vi "SwapAndFormat.vi"(4 "Mode Index":i32=2, 6 "Undo pointer":i32, 7 "Layout Ref":refnum<vi>, 8 "error in (no error)":errorcluster, 9 "Table CtlRef In":refnum<vi>, 10 "Col Array in":refnum<class "Column.lvclass">[](array[class]), 11 "OldTable Array in":T1) -> (0 "error out":errorcluster, 3 "OldTable Array out":T1)   [LabVIEW 2013]
doc: "Original use was in Un(Re)doTblChng.vi. It can also be used to apply (block-wise) changes to the table (as with PasteSafe.vi) with best choices for formatting. Input new table as 1st element in an array of cluster of table and set undo pointer to zero."
uses:
  TypeDefs/TableArray.ctl
  ColumnVIs/Column/Column.lvclass
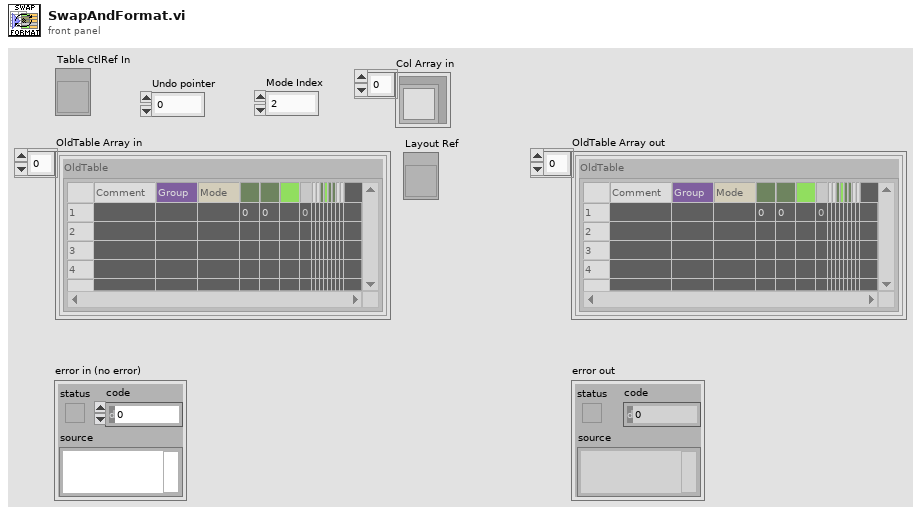
[diagram p1: front panel]
types:
  T1 = typedef "TableArray.ctl" = cluster{"OldTable":string[][]}[]
  T2 = typedef "LVRowAndColumnTypeDef.ctl" = cluster{"Row":i32, "Column":i32}
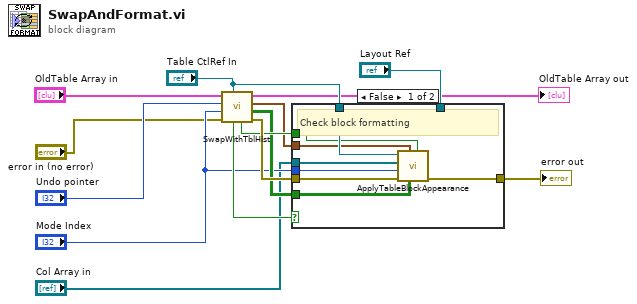
[diagram p0: block diagram]
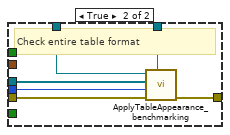
[diagram p2: hidden frame]
diagram:
  n1 = call "SwapWithTblHist.vi"("Table CtlRef In"="Table CtlRef In", "error in (no error)"="error in (no error)", "Mode Index"="Mode Index", "Undo pointer"="Undo pointer", "OldTable Array in"="OldTable Array in") -> ("error out"=w14:errorcluster, "changed? subarray"=w11:bool[][], "Change start"=w10:T2, "OldTable Array out"=→"OldTable Array out":T1, "Mode change?"=w12:bool, "Size mismatch?"=w13:bool)  [unwired: 1 in]
  n2 = case shown="False" w13 {
    tunnel: w14 -> [w22 w28]
    tunnel: [w21 w27] -> w2
    tunnel: "Table CtlRef In" -> [w20 w26]
    tunnel: "Layout Ref" -> [_ w25]
    tunnel: "Col Array in" -> [w19 w24]
    tunnel: "Mode Index" -> [w18 w23]
    tunnel: w12 -> [w17 _]
    tunnel: w11 -> [w16 _]
    tunnel: w10 -> [w15 _]
    frame False {
      # "Check block formatting"
      n3 = call "ApplyTableBlockAppearance.vi"("Check Mode?"=w17, "changed? subarray"=w16, "Change start"=w15, "error in (no error)"=w22, "Mode Index"=w18, "Col Array in"=w19, "Table Ref in"=w20) -> ("error out"=w21:errorcluster)  [unwired: 4 in]
    }
    frame True {
      # "Check entire table format"
      n4 = call "ApplyTableAppearance_benchmarking.vi"("Layout Ring Ref"=w25, "error in (no error)"=w28, "Mode Index"=w23, "Col Array in"=w24, "Table Ref in"=w26) -> ("error out"=w27:errorcluster)  [unwired: 5 in, 1 out]
    }
  }
  "error out" <- w2
